vi "Add Rx Transfer Configuration.vi"(8 "error in":errorcluster, 10 "configuration":T1, 11 "transfer":T2={"core"={"name"="Transfer"}, "component settings"=[], "channels"=[]} {"channels"."core"."string offset" format="%d bytes"}) -> (0 "error out":errorcluster, 3 "transfer out":T2={"core"={"name"="Transfer"}, "component settings"=[], "channels"=[]} {"channels"."core"."string offset" format="%d bytes"})   [LabVIEW 2020, in "DSF UDP Configuration API.lvlib"]
uses:
  DSF UDP Configuration API.lvlib
  <vilib>/addons/VeriStand Custom Device Scripting APIs/Data Sharing Framework/DSF Core.lvlibp/Typedefs/DSF Engine Transfer Configuration.ctl
  <vilib>/addons/VeriStand Custom Device Scripting APIs/Data Sharing Framework/DSF Core.lvlibp/Typedefs/Core Transfer Configuration.ctl
  <vilib>/addons/VeriStand Custom Device Scripting APIs/Data Sharing Framework/DSF Core.lvlibp/Typedefs/DSF Settings Info.ctl
  <vilib>/addons/VeriStand Custom Device Scripting APIs/Data Sharing Framework/DSF Core.lvlibp/Typedefs/DSF Engine Channel Configuration.ctl
  <vilib>/addons/VeriStand Custom Device Scripting APIs/Data Sharing Framework/DSF Core.lvlibp/Typedefs/Core Channel Configuration.ctl
  <vilib>/addons/VeriStand Custom Device Scripting APIs/Data Sharing Framework/DSF Core.lvlibp/Typedefs/DSF Data Type.ctl
  Types/Rx Configuration.ctl
  357240c7-7acf-4cfc-919d-c046660ecadf.vi
  <vilib>/addons/VeriStand Custom Device Scripting APIs/Data Sharing Framework/DSF Core.lvlibp
  <vilib>/addons/VeriStand Custom Device Scripting APIs/Data Sharing Framework/DSF Core.lvlibp/Classes/Configuration/Core/Transfer/Transfer Configuration.lvclass
  <vilib>/addons/VeriStand Custom Device Scripting APIs/Data Sharing Framework/DSF Core.lvlibp/Classes/Configuration/Core/Channel/Channel Configuration.lvclass
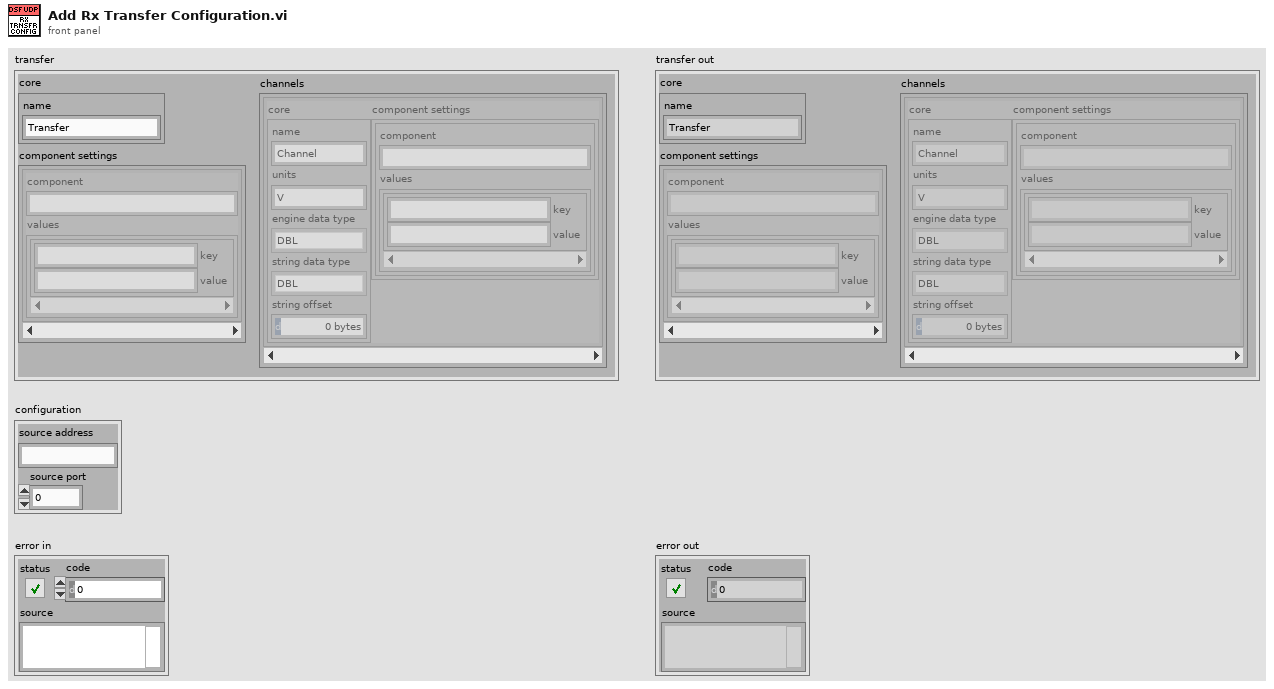
[diagram p1: front panel]
types:
  T1 = typedef "DSF UDP Configuration API.lvlib/Rx Configuration.ctl" = cluster{"source address":string, "source port":u16}
  T2 = typedef "DSF Core.lvlibp/DSF Engine Transfer Configuration.ctl" = cluster{"core":T3, "component settings":T4[], "channels":T5[]}
  T3 = typedef "DSF Core.lvlibp/Transfer Configuration.lvclass/Core Transfer Configuration.ctl" = cluster{"name":string}
  T4 = typedef "DSF Core.lvlibp/DSF Settings Info.ctl" = cluster{"component":string, "values":cluster{"key":string, "value":string}[]}
  T5 = typedef "DSF Core.lvlibp/DSF Engine Channel Configuration.ctl" = cluster{"core":T6, "component settings":T4[]}
  T6 = typedef "DSF Core.lvlibp/Channel Configuration.lvclass/Core Channel Configuration.ctl" = cluster{"name":string, "units":string, "engine data type":T7, "string data type":T7, "string offset":u64}
  T7 = typedef "DSF Core.lvlibp/DSF Data Type.ctl" = enum8{"Bool", "SGL", "DBL", "I8", "I16", "I32", "I64", "U8", "U16", "U32", "U64"}
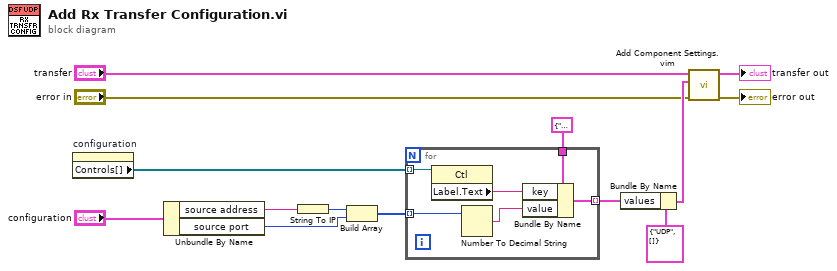
[diagram p0: block diagram]
diagram:
  n1 = property on="configuration" class="Clust (strict)"() -> ("Controls[]"=w14:refnum<vi>[])  [unwired: 2 in, 2 out]
  n2 = Unbundle By Name("configuration") -> ("source address"=w12:string, "source port"=w10:u16)
  n3 = String To IP(1:w12) -> (0:w11:u32)
  n4 = Build Array(w11, w10) -> (w9:u32[])
  n5 = for {
    tunnel: w14 -> [w20] mode=indexing
    tunnel: w9 -> [w19] mode=indexing
    tunnel: cluster{"key":string, "value":string} {"key"="", "value"=""} ("setting") -> [w18]
    tunnel: [w15] -> w6 mode=indexing
    n6 = property class="Ctl"(reference=w20) -> ("Label.Text"=w17:string)  [unwired: 1 in, 2 out]
    n7 = Number To Decimal String(number=w19) -> (decimal integer string=w16:string)  [unwired: 1 in]
    n8 = Bundle By Name(cluster=w18, "key"=w17, "value"=w16) -> (w15:cluster{"key":string, "value":string})
  }
  n9 = Bundle By Name(cluster=T4 {"component"="UDP", "values"=[]} ("component settings"), "values"=w6) -> (w4:T4)
  n10 = call "Add Component Settings.vim"("error in"="error in", "component settings"=w4, "dsf configuration"="transfer") -> ("error out"=→"error out":errorcluster, "dsf configuration out"=→"transfer out":T2)  [unwired: 7 in]
